vi "RT_RK4_rotation (SubVI).vi"(8 "dt":dbl, 9 "dt*0.5":dbl, 10 "H(i)":dbl[](array[numeric]), 11 "ang_acc":dbl[](array[numeric])) -> (0 "W_b(i+1)":dbl[](array[numeric]), 1 "W(i+1)":dbl[](array[numeric]), 2 "q(i+1)":dbl[](array[numeric]), 3 "H(i+1)":dbl[](array[numeric]))   [LabVIEW 2011]
uses:
  <vilib>/Analysis/Matrix/NI_Matrix.lvlib
  <vilib>/Analysis/NI_AALBase.lvlib
  <vilib>/Analysis/Matrix/Numeric/Conversions/Matrix To Array - RM.vi
  <vilib>/Analysis/Matrix/Numeric/Conversions/Array To Matrix - RA2.vi
  <vilib>/Analysis/baseanly.llb/Real A x B.vi
  <vilib>/Analysis/Matrix/Numeric/Conversions/Array To Matrix - RA.vi
  <vilib>/Analysis/NI_AALPro.lvlib
  <vilib>/Analysis/_algsub.llb/Real Vector Norm.vi
  <vilib>/Analysis/_algsub.llb/Vector Norm Type.ctl
panel:
  out "x+y":dbl[](array[numeric])
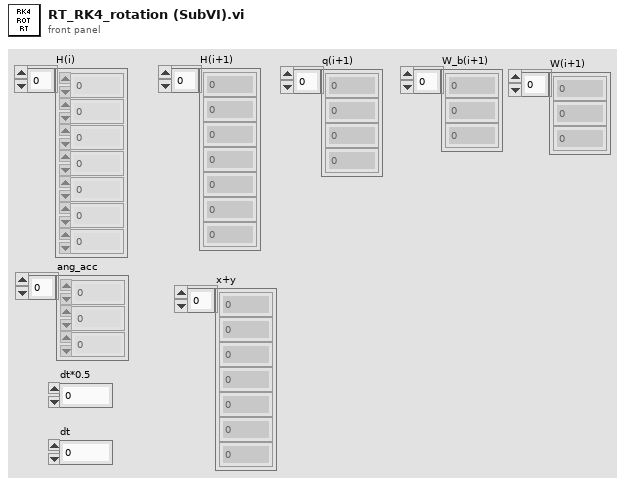
[diagram p1: front panel]
types:
  T1 = typedef "NI_AALPro.lvlib/Vector Norm Type.ctl" = u16
  T2 = typedef "NI_Matrix.lvlib/RealMatrix.ctl" = dbl[][]
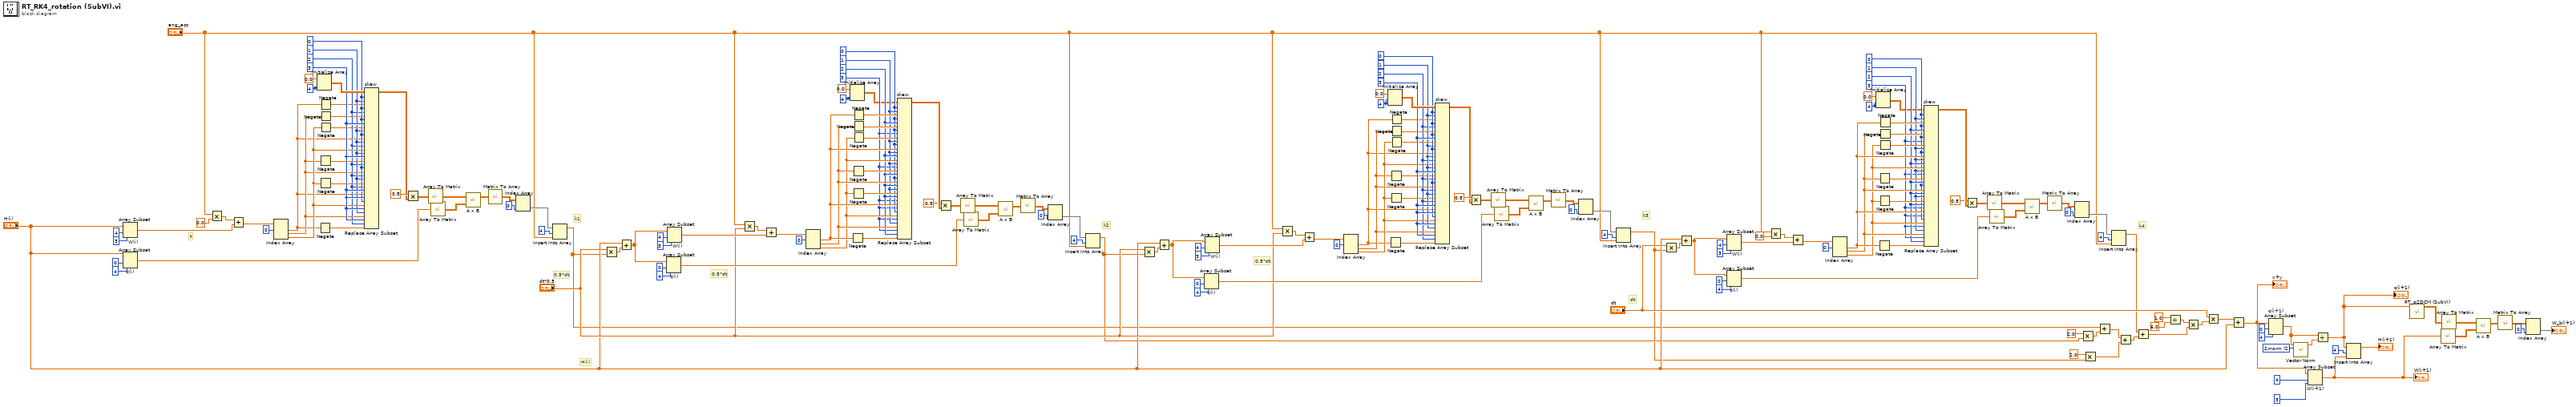
[diagram p0: block diagram]
diagram:
  w19 = T1 2 items=["1-norm"=1, "2-norm"=2, "Inf-norm"=3, "-Inf-norm"=4, "User Defined"=5] ("norm type")
  w34 = 3 ("index (col)")
  w37 = 2 ("index (row)")
  w36 = 1 ("index (col)")
  w35 = 0 ("index (row)")
  w4 = 4 ("dimension size")
  w98 = 3 ("index (col)")
  w95 = 2 ("index (row)")
  w96 = 1 ("index (col)")
  w97 = 0 ("index (row)")
  w3 = 4 ("dimension size")
  w108 = 3 ("index (col)")
  w111 = 2 ("index (row)")
  w110 = 1 ("index (col)")
  w109 = 0 ("index (row)")
  w106 = 4 ("dimension size")
  w169 = 3 ("index (col)")
  w166 = 2 ("index (row)")
  w167 = 1 ("index (col)")
  w168 = 0 ("index (row)")
  w171 = 4 ("dimension size")
  # "dt"
  # "0.5*dt"
  # "k4"
  # "0.5*dt"
  # "0.5*dt"
  # "H(i)"
  # "k3"
  # "t"
  # "k2"
  # "k1"
  n1 = Array Subset "q(i)"(array="H(i)", index=0, length=4) -> (w146:dbl[])
  n2 = Array Subset "W(i)"(array="H(i)", index=4, length=3) -> (w161:dbl[])
  n3 = Multiply(x="ang_acc", y=0.0) -> (x*y=w173:dbl[])
  n4 = Add(x=w173, y=w161) -> (x+y=w160:dbl[])
  n5 = Index Array(array=w160, index #1=0 ("index")) -> (element #1=w150:dbl, element #2=w151:dbl, element #3=w152:dbl)  [unwired: 2 in]
  n6 = Initialize Array(0.0 ("element"), w171, w171) -> (w170:dbl[][])
  n7 = Negate(x=w150) -> (-x=w153:dbl)
  n8 = Negate(x=w151) -> (-x=w155:dbl)
  n9 = Negate(x=w152) -> (-x=w154:dbl)
  n10 = Negate(x=w150) -> (-x=w158:dbl)
  n11 = Negate(x=w151) -> (-x=w157:dbl)
  n12 = Negate(x=w152) -> (-x=w156:dbl)
  n13 = Replace Array Subset "skew"(array=w170, new element #1=w158, index (row) #1=w168, index (col) #1=w167, new element #2=w157, index (row) #2=w168, index (col) #2=w166, new element #3=w156, index (row) #3=w168, index (col) #3=w169, new element #4=w150, index (row) #4=w167, index (col) #4=w168, new element #5=w152, index (row) #5=w167, index (col) #5=w166, new element #6=w155, index (row) #6=w167, index (col) #6=w169, new element #7=w151, index (row) #7=w166, index (col) #7=w168, new element #8=w154, index (row) #8=w166, index (col) #8=w167, new element #9=w150, index (row) #9=w166, index (col) #9=w169, new element #10=w152, index (row) #10=w169, index (col) #10=w168, new element #11=w151, index (row) #11=w169, index (col) #11=w167, new element #12=w153, index (row) #12=w169, index (col) #12=w166) -> (w148:dbl[][])
  n14 = Multiply(x=0.5, y=w148) -> (x*y=w147:dbl[][])
  n15 = call-poly <vilib>:"Array To Matrix.vi"("Real 2D Array"=w147) -> ("Real Matrix"=w145:T2)
  n16 = call-poly <vilib>:"Array To Matrix.vi"("Real 1D Array"=w146) -> ("Real Matrix (Column Vector)"=w144:T2)
  n17 = call-poly <vilib>:"A x B.vi"("B"=w144, "A"=w145) -> ("A x B"=w142:T2)  [unwired: 1 out]
  n18 = call-poly <vilib>:"Matrix To Array.vi"("Real Matrix"=w142) -> ("Real 2D Array"=w143:dbl[][])
  n19 = Index Array(array=w143, index (col)=0 ("index (row)")) -> (element=w141:dbl[])  [unwired: 1 in]
  n20 = Insert Into Array(array=w141, index=4, new element="ang_acc") -> (w24:dbl[])
  n21 = Multiply(x="dt*0.5", y=w24) -> (x*y=w175:dbl[])
  n22 = Add(x="H(i)", y=w175) -> (x+y=w103:dbl[])
  n23 = Array Subset "q(i)"(array=w103, index=0, length=4) -> (w131:dbl[])
  n24 = Array Subset "W(i)"(array=w103, index=4, length=3) -> (w116:dbl[])
  n25 = Multiply(x="ang_acc", y="dt*0.5") -> (x*y=w104:dbl[])
  n26 = Add(x=w104, y=w116) -> (x+y=w117:dbl[])
  n27 = Index Array(array=w117, index #1=0 ("index")) -> (element #1=w127:dbl, element #2=w126:dbl, element #3=w125:dbl)  [unwired: 2 in]
  n28 = Initialize Array(0.0 ("element"), w106, w106) -> (w107:dbl[][])
  n29 = Negate(x=w127) -> (-x=w124:dbl)
  n30 = Negate(x=w126) -> (-x=w122:dbl)
  n31 = Negate(x=w125) -> (-x=w123:dbl)
  n32 = Negate(x=w127) -> (-x=w119:dbl)
  n33 = Negate(x=w126) -> (-x=w120:dbl)
  n34 = Negate(x=w125) -> (-x=w121:dbl)
  n35 = Replace Array Subset "skew"(array=w107, new element #1=w119, index (row) #1=w109, index (col) #1=w110, new element #2=w120, index (row) #2=w109, index (col) #2=w111, new element #3=w121, index (row) #3=w109, index (col) #3=w108, new element #4=w127, index (row) #4=w110, index (col) #4=w109, new element #5=w125, index (row) #5=w110, index (col) #5=w111, new element #6=w122, index (row) #6=w110, index (col) #6=w108, new element #7=w126, index (row) #7=w111, index (col) #7=w109, new element #8=w123, index (row) #8=w111, index (col) #8=w110, new element #9=w127, index (row) #9=w111, index (col) #9=w108, new element #10=w125, index (row) #10=w108, index (col) #10=w109, new element #11=w126, index (row) #11=w108, index (col) #11=w110, new element #12=w124, index (row) #12=w108, index (col) #12=w111) -> (w129:dbl[][])
  n36 = Multiply(x=0.5, y=w129) -> (x*y=w130:dbl[][])
  n37 = call-poly <vilib>:"Array To Matrix.vi"("Real 2D Array"=w130) -> ("Real Matrix"=w132:T2)
  n38 = call-poly <vilib>:"Array To Matrix.vi"("Real 1D Array"=w131) -> ("Real Matrix (Column Vector)"=w133:T2)
  n39 = call-poly <vilib>:"A x B.vi"("B"=w133, "A"=w132) -> ("A x B"=w135:T2)  [unwired: 1 out]
  n40 = call-poly <vilib>:"Matrix To Array.vi"("Real Matrix"=w135) -> ("Real 2D Array"=w134:dbl[][])
  n41 = Index Array(array=w134, index (col)=0 ("index (row)")) -> (element=w136:dbl[])  [unwired: 1 in]
  n42 = Insert Into Array(array=w136, index=4, new element="ang_acc") -> (w23:dbl[])
  n43 = Multiply(x="dt*0.5", y=w23) -> (x*y=w67:dbl[])
  n44 = Add(x="H(i)", y=w67) -> (x+y=w102:dbl[])
  n45 = Array Subset "q(i)"(array=w102, index=0, length=4) -> (w75:dbl[])
  n46 = Array Subset "W(i)"(array=w102, index=4, length=3) -> (w90:dbl[])
  n47 = Multiply(x="ang_acc", y="dt*0.5") -> (x*y=w101:dbl[])
  n48 = Add(x=w101, y=w90) -> (x+y=w89:dbl[])
  n49 = Index Array(array=w89, index #1=0 ("index")) -> (element #1=w79:dbl, element #2=w80:dbl, element #3=w81:dbl)  [unwired: 2 in]
  n50 = Initialize Array(0.0 ("element"), w3, w3) -> (w99:dbl[][])
  n51 = Negate(x=w79) -> (-x=w82:dbl)
  n52 = Negate(x=w80) -> (-x=w84:dbl)
  n53 = Negate(x=w81) -> (-x=w83:dbl)
  n54 = Negate(x=w79) -> (-x=w87:dbl)
  n55 = Negate(x=w80) -> (-x=w86:dbl)
  n56 = Negate(x=w81) -> (-x=w85:dbl)
  n57 = Replace Array Subset "skew"(array=w99, new element #1=w87, index (row) #1=w97, index (col) #1=w96, new element #2=w86, index (row) #2=w97, index (col) #2=w95, new element #3=w85, index (row) #3=w97, index (col) #3=w98, new element #4=w79, index (row) #4=w96, index (col) #4=w97, new element #5=w81, index (row) #5=w96, index (col) #5=w95, new element #6=w84, index (row) #6=w96, index (col) #6=w98, new element #7=w80, index (row) #7=w95, index (col) #7=w97, new element #8=w83, index (row) #8=w95, index (col) #8=w96, new element #9=w79, index (row) #9=w95, index (col) #9=w98, new element #10=w81, index (row) #10=w98, index (col) #10=w97, new element #11=w80, index (row) #11=w98, index (col) #11=w96, new element #12=w82, index (row) #12=w98, index (col) #12=w95) -> (w77:dbl[][])
  n58 = Multiply(x=0.5, y=w77) -> (x*y=w76:dbl[][])
  n59 = call-poly <vilib>:"Array To Matrix.vi"("Real 2D Array"=w76) -> ("Real Matrix"=w74:T2)
  n60 = call-poly <vilib>:"Array To Matrix.vi"("Real 1D Array"=w75) -> ("Real Matrix (Column Vector)"=w73:T2)
  n61 = call-poly <vilib>:"A x B.vi"("B"=w73, "A"=w74) -> ("A x B"=w71:T2)  [unwired: 1 out]
  n62 = call-poly <vilib>:"Matrix To Array.vi"("Real Matrix"=w71) -> ("Real 2D Array"=w72:dbl[][])
  n63 = Index Array(array=w72, index (col)=0 ("index (row)")) -> (element=w70:dbl[])  [unwired: 1 in]
  n64 = Insert Into Array(array=w70, index=4, new element="ang_acc") -> (w22:dbl[])
  n65 = Multiply(x="dt", y=w22) -> (x*y=w65:dbl[])
  n66 = Add(x="H(i)", y=w65) -> (x+y=w30:dbl[])
  n67 = Array Subset "q(i)"(array=w30, index=0, length=4) -> (w57:dbl[])
  n68 = Array Subset "W(i)"(array=w30, index=4, length=3) -> (w42:dbl[])
  n69 = Multiply(x="ang_acc", y=0.0) -> (x*y=w31:dbl[])
  n70 = Add(x=w31, y=w42) -> (x+y=w43:dbl[])
  n71 = Index Array(array=w43, index #1=0 ("index")) -> (element #1=w53:dbl, element #2=w52:dbl, element #3=w51:dbl)  [unwired: 2 in]
  n72 = Initialize Array(0.0 ("element"), w4, w4) -> (w33:dbl[][])
  n73 = Negate(x=w53) -> (-x=w50:dbl)
  n74 = Negate(x=w52) -> (-x=w48:dbl)
  n75 = Negate(x=w51) -> (-x=w49:dbl)
  n76 = Negate(x=w53) -> (-x=w45:dbl)
  n77 = Negate(x=w52) -> (-x=w46:dbl)
  n78 = Negate(x=w51) -> (-x=w47:dbl)
  n79 = Replace Array Subset "skew"(array=w33, new element #1=w45, index (row) #1=w35, index (col) #1=w36, new element #2=w46, index (row) #2=w35, index (col) #2=w37, new element #3=w47, index (row) #3=w35, index (col) #3=w34, new element #4=w53, index (row) #4=w36, index (col) #4=w35, new element #5=w51, index (row) #5=w36, index (col) #5=w37, new element #6=w48, index (row) #6=w36, index (col) #6=w34, new element #7=w52, index (row) #7=w37, index (col) #7=w35, new element #8=w49, index (row) #8=w37, index (col) #8=w36, new element #9=w53, index (row) #9=w37, index (col) #9=w34, new element #10=w51, index (row) #10=w34, index (col) #10=w35, new element #11=w52, index (row) #11=w34, index (col) #11=w36, new element #12=w50, index (row) #12=w34, index (col) #12=w37) -> (w55:dbl[][])
  n80 = Multiply(x=0.5, y=w55) -> (x*y=w56:dbl[][])
  n81 = call-poly <vilib>:"Array To Matrix.vi"("Real 2D Array"=w56) -> ("Real Matrix"=w58:T2)
  n82 = call-poly <vilib>:"Array To Matrix.vi"("Real 1D Array"=w57) -> ("Real Matrix (Column Vector)"=w59:T2)
  n83 = call-poly <vilib>:"A x B.vi"("B"=w59, "A"=w58) -> ("A x B"=w61:T2)  [unwired: 1 out]
  n84 = call-poly <vilib>:"Matrix To Array.vi"("Real Matrix"=w61) -> ("Real 2D Array"=w60:dbl[][])
  n85 = Index Array(array=w60, index (col)=0 ("index (row)")) -> (element=w62:dbl[])  [unwired: 1 in]
  n86 = Multiply(x=2.0, y=w23) -> (x*y=w179:dbl[])
  n87 = Multiply(x=2.0, y=w22) -> (x*y=w183:dbl[])
  n88 = Add(x=w24, y=w179) -> (x+y=w181:dbl[])
  n89 = Insert Into Array(array=w62, index=4, new element="ang_acc") -> (w25:dbl[])
  n90 = Add(x=w181, y=w183) -> (x+y=w184:dbl[])
  n91 = Add(x=w25, y=w184) -> (x+y=w185:dbl[])
  n92 = Divide(x=1.0, y=6.0) -> (x/y=w178:dbl)
  n93 = Multiply(x=w178, y=w185) -> (x*y=w186:dbl[])
  n94 = Multiply(x="dt", y=w186) -> (x*y=w187:dbl[])
  n95 = Add(x=w187, y="H(i)") -> (x+y=w6:dbl[])
  "x+y" <- w6
  n96 = Array Subset "q(i+1)"(array=w6, index=0, length=4) -> (w18:dbl[])
  n97 = call-poly <vilib>:"Vector Norm.vi"("norm type"=w19, "Input Vector"=w18) -> ("norm"=w17:dbl)  [unwired: 8 in, 1 out]
  n98 = Array Subset "W(i+1)"(array=w6, index=4, length=3) -> (w5:dbl[])
  "W(i+1)" <- w5
  n99 = Divide(x=w18, y=w17) -> (x/y=w14:dbl[])
  "q(i+1)" <- w14
  n100 = Insert Into Array(array=w14, index=4, new element=w5) -> (→"H(i+1)":dbl[])
  n101 = call "RT_q2DCM (SubVI).vi"("Quaternion"=w14) -> ("DCM"=w9:dbl[][])  [unwired: 10 in]
  n102 = call-poly <vilib>:"Array To Matrix.vi"("Real 1D Array"=w5) -> ("Real Matrix (Column Vector)"=w10:T2)
  n103 = call-poly <vilib>:"Array To Matrix.vi"("Real 2D Array"=w9) -> ("Real Matrix"=w8:T2)
  n104 = call-poly <vilib>:"A x B.vi"("B"=w10, "A"=w8) -> ("A x B"=w12:T2)  [unwired: 1 out]
  n105 = call-poly <vilib>:"Matrix To Array.vi"("Real Matrix"=w12) -> ("Real 2D Array"=w11:dbl[][])
  n106 = Index Array(array=w11, index (col)=0 ("index (row)")) -> (element=→"W_b(i+1)":dbl[])  [unwired: 1 in]
